vi "Pop.vi"() -> ()   [LabVIEW 2024, in "POTCircularBuffer.Tests.Units.lvlib"]
uses:
  POTCircularBuffer.Tests.Units.lvlib
  TypedCircularBuffer/Type.ctl
  Type.ctl
  POTTypedCircularBuffer.lvclass
  POTTypedCircularBuffer.lvclass/POTTypedCircularBuffer.ctl
  Wrap.vi
  ReadCount.vi
  Reorder.vi
  IsEmpty.vi
  <vilib>/addons/_JKI Toolkits/Caraya/classes/Assert/Assert Equal Value_Variant.vi
  <vilib>/addons/_JKI Toolkits/Caraya/classes/Assert/Assert False.vi
  <vilib>/addons/_JKI Toolkits/Caraya/classes/Assert/Assert.lvclass
  <vilib>/addons/_JKI Toolkits/Caraya/classes/Test/Test.lvclass
  TypedCircularBuffer/TypedCircularBuffer.lvclass
panel:
  out "POTTypedCircularBuffer out":refnum<class "POTTypedCircularBuffer.lvclass">
  in  "expected":T1[](array[typedef])=[2, 3, 4, 5, 6, 7, 8]
  out "peaked":T2[](array[typedef])
  out "element":T1
  out "Flushed Buffer":T1[](array[typedef])
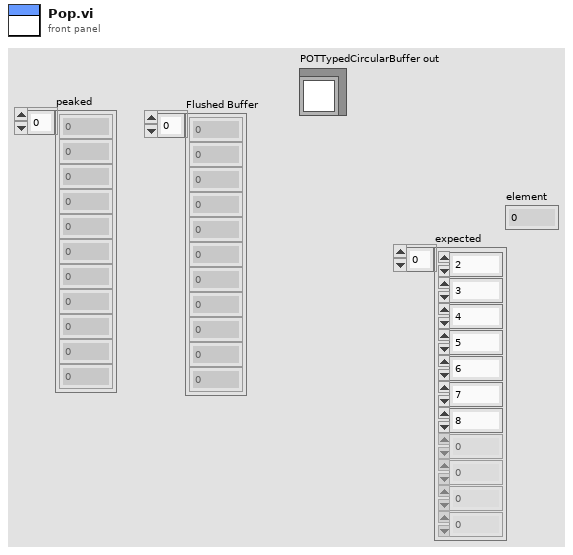
[diagram p1: front panel]
types:
  T1 = typedef "TypedCircularBuffer.lvclass/Type.ctl" = i32
  T2 = typedef "POTTypedCircularBuffer.lvclass/Type.ctl" = i32
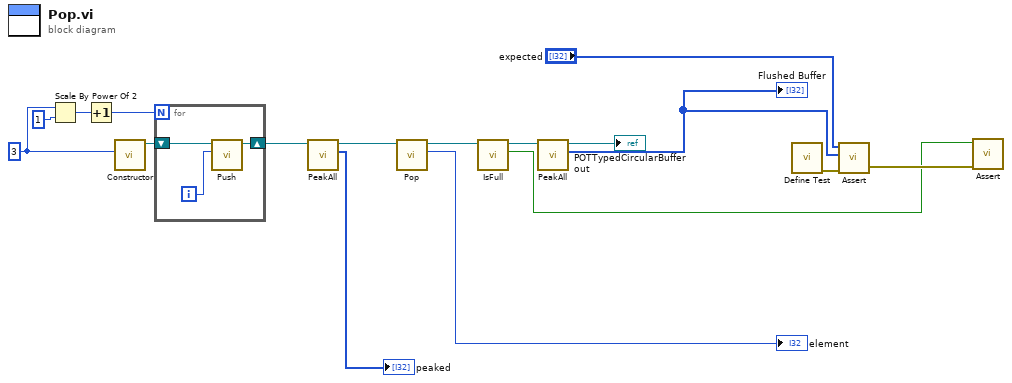
[diagram p0: block diagram]
diagram:
  w8 = u32 3 ("Capacity")
  n1 = Scale By Power Of 2(n=w8, x=1) -> (x*2^n=w10:i32)
  n2 = Increment(x=w10) -> (x+1=w9:i32)
  n3 = call "Constructor.vi"("Capacity 2^n"=w8) -> ("POTTypedCircularBuffer out"=w15:refnum<class "POTTypedCircularBuffer.lvclass">)  [unwired: 10 in]
  n4 = for {
    N: w9 -> [_]
    shift-right: [w19] -> w7
    shift-left: w15 -> [w20]
    i -> [w18]
    n5 = call "Push.vi"("Element"=w18, "POTTypedCircularBuffer in"=w20) -> ("POTTypedCircularBuffer out"=w19:refnum<class "POTTypedCircularBuffer.lvclass">)  [unwired: 9 in]
  }
  n6 = call "PeakAll.vi"("POTTypedCircularBuffer in"=w7) -> ("Copied Buffer"=→"peaked":T2[], "POTTypedCircularBuffer out"=w6:refnum<class "POTTypedCircularBuffer.lvclass">)  [unwired: 9 in]
  n7 = call "Pop.vi"("POTTypedCircularBuffer in"=w6) -> ("element"=→"element":T2, "POTTypedCircularBuffer out"=w13:refnum<class "POTTypedCircularBuffer.lvclass">)  [unwired: 8 in, 1 out]
  n8 = call "IsFull.vi"("POTTypedCircularBuffer in"=w13) -> ("Full?"=w2:bool, "POTTypedCircularBuffer out"=w12:refnum<class "POTTypedCircularBuffer.lvclass">)  [unwired: 9 in]
  n9 = call "PeakAll.vi"("POTTypedCircularBuffer in"=w12) -> ("Copied Buffer"=w3:T2[], "POTTypedCircularBuffer out"=→"POTTypedCircularBuffer out":refnum<class "POTTypedCircularBuffer.lvclass">)  [unwired: 9 in]
  "Flushed Buffer" <- w3
  n10 = call <vilib>:"Define Test.vi"() -> ("error out"=w17:errorcluster)  [unwired: 10 in, 1 out]
  n11 = call-poly <vilib>:"Assert.vi"("error in (no error)"=w17, "Y"=w3, "X"="expected") -> ("error out"=w16:errorcluster)  [unwired: 7 in, 1 out]
  n12 = call-poly <vilib>:"Assert.vi"("error in (no error)"=w16, "False?"=w2) -> ()  [unwired: 8 in, 2 out]
